vi "_GetData_I32.vi"(8 "Error In":errorcluster, 10 "Index":i32=-1, 11 "ByteBuffer In":refnum<class "ByteBuffer.lvclass">) -> (0 "Error Out":errorcluster, 2 "Data":i32, 3 "ByteBuffer Out":refnum<class "ByteBuffer.lvclass">)   [LabVIEW 2015, in "ByteBuffer.lvclass"]
uses:
  ByteBuffer.lvclass
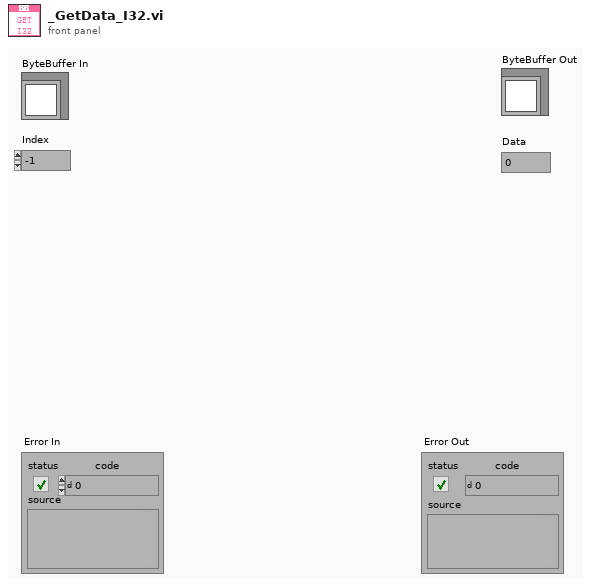
[diagram p1: front panel]
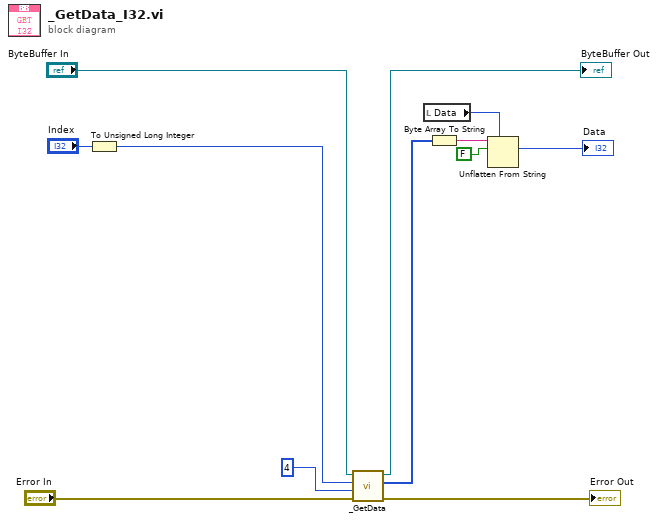
[diagram p0: block diagram]
diagram:
  n1 = To Unsigned Long Integer(number="Index") -> (unsigned 32bit integer=w7:u32)
  n2 = call "_GetData.vi"("Error In"="Error In", "Length"=4, "Index Or Position"=w7, "ByteBuffer In"="ByteBuffer In") -> ("Error Out"=→"Error Out":errorcluster, "Byte Array"=w4:u8[], "ByteBuffer Out"=→"ByteBuffer Out":refnum<class "ByteBuffer.lvclass">)  [unwired: 5 in]
  n3 = local read "Data"() -> (w5:i32)
  n4 = Byte Array To String(unsigned byte array=w4) -> (string=w3:string)
  n5 = Unflatten From String(type=w5, binary string=w3, data includes array or string size? (T)=FALSE) -> (value=→"Data":i32)  [unwired: 2 in, 2 out]
